vi "Set id type as none.vi"(8 "error in (no error)":errorcluster, 11 "id in":refnum<class "id.lvclass">) -> (0 "error out":errorcluster, 3 "id out":refnum<class "id.lvclass">)   [LabVIEW 2015, in "id.lvclass"]
uses:
  id.lvclass
  id.lvclass/id.ctl
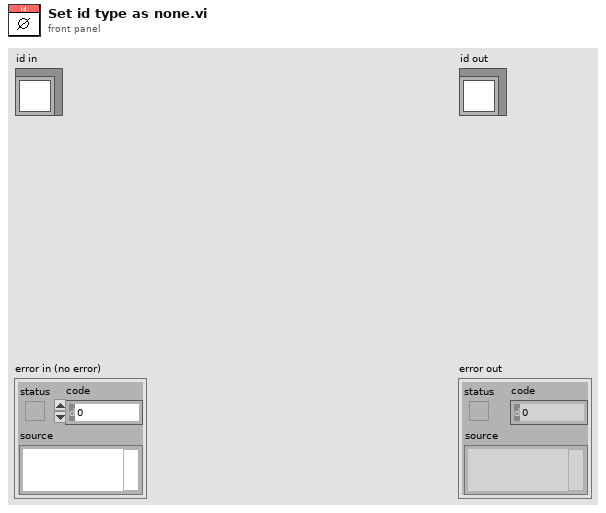
[diagram p1: front panel]
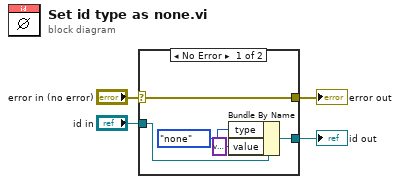
[diagram p0: block diagram]
diagram:
  n1 = case shown="No Error" "error in (no error)" {
    selector: "error in (no error)" -> [w6 w11]
    tunnel: [w6 w11] -> w3
    tunnel: [w7 w10] -> w1
    tunnel: "id in" -> [w9 w10]
    frame No Error {
      n2 = Bundle By Name(cluster=w9, "type"=enum16{"none", "String", "Number", "NULL"}."none", "value"=variant) -> (w7:refnum<class "id.lvclass">)
    }
    frame Error {
    }
  }
  "error out" <- w3
  "id out" <- w1
